vi "Demo.vi"() -> ()   [LabVIEW 2021, in "Ring Buffer Time Series Data.lvlib"]
uses:
  Ring Buffer Time Series Data.lvlib
  SubVIs/Split Values Array.vi
  SubVIs/Replace Values Array Multiple Timestamps.vi
  SubVIs/Rotate Buffer.vi
  SubVIs/Newest Value Index.vi
  SubVIs/empty buffer check.vi
  SubVIs/Replace Values Array One Timestamp.vi
  SubVIs/Enforce array size one timestamp.vi
  SubVIs/Enforce array size multiple timestamps.vi
panel:
  out "empty buffer? (previous)":bool
  out "empty buffer? (latest)":bool
  out "empty buffer?":bool
  out "v-latest 3":u8[](array[numeric])
  out "v-latest 2":u8[](array[numeric])
  out "t-latest 3":u64
  out "t-latest 2":u64
  out "Value changed? 2":bool
  out "Value changed?":bool
  out "v3":u8[](array[numeric])
  out "t3":u64[](array[numeric])
  out "v1":u8[](array[numeric])
  out "t1":u64[](array[numeric])
  out "v-latest":u8[](array[numeric])
  out "t-latest":u64
  out "t2":u64[](array[numeric])
  out "v2":u8[](array[numeric])
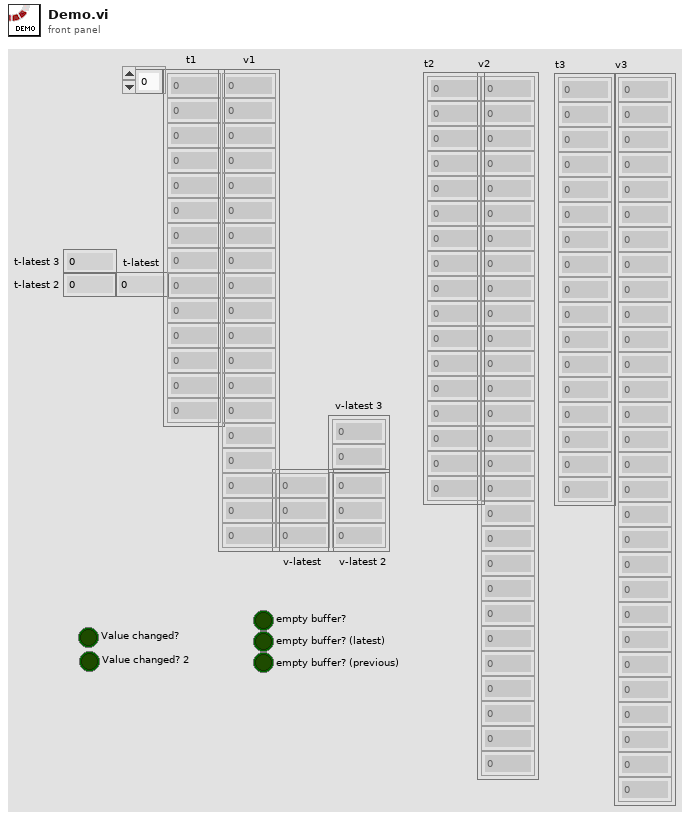
[diagram p1: front panel]
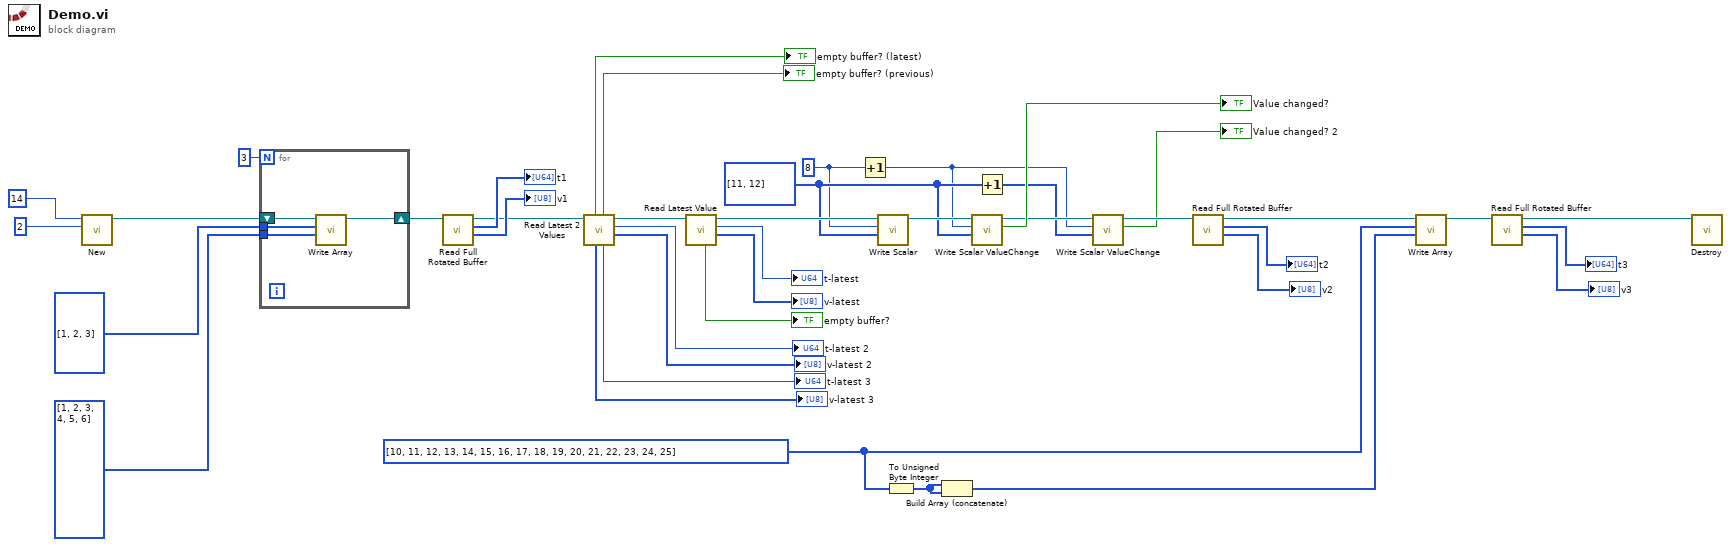
[diagram p0: block diagram]
diagram:
  w26 = u64[] [10, 11, 12, 13, 14, 15, 16, 17, 18, 19, 20, 21, 22, 23, 24, 25] ("Timestamps")
  w14 = u8[] [11, 12] ("Data")
  w12 = u64 8 ("Timestamp")
  n1 = call "New.vi"("#bytes per timestamp"=2 ("#bytes per value"), "Buffer Size (#timestamps)"=14 ("Buffer Size")) -> ("Ring buffer DVR"=w1:refnum<data-value>)  [unwired: 8 in, 1 out]
  n2 = for {
    N: 3 -> [_]
    tunnel: u8[] [1, 2, 3, 4, 5, 6] ("Timestamps") -> [w43]
    tunnel: u64[] [1, 2, 3] ("Timestamps") -> [w41]
    shift-right: [w42] -> w39
    shift-left: w1 -> [w44]
    n3 = call "Write Array.vi"("Data"=w43, "Timestamps"=w41, "Ring buffer DVR in"=w44) -> ("Ring buffer DVR out"=w42:refnum<data-value>)  [unwired: 7 in, 1 out]
  }
  n4 = call "Read Full Rotated Buffer.vi"("Ring buffer DVR in"=w39) -> ("Values"=→"v1":u8[], "Timestamps"=→"t1":u64[], "Ring buffer DVR out"=w10:refnum<data-value>)  [unwired: 5 in, 3 out]
  n5 = call "Read Latest 2 Values.vi"("Ring buffer DVR in"=w10) -> ("Values (latest)"=→"v-latest 2":u8[], "Timestamp (latest)"=→"t-latest 2":u64, "Ring buffer DVR out"=w9:refnum<data-value>, "Timestamp (previous)"=→"t-latest 3":u64, "empty buffer? (previous)"=→"empty buffer? (previous)":bool, "Values (previous)"=→"v-latest 3":u8[], "empty buffer? (latest)"=→"empty buffer? (latest)":bool)  [unwired: 3 in, 1 out]
  n6 = call "Read Latest Value.vi"("Ring buffer DVR in"=w9) -> ("Values"=→"v-latest":u8[], "Timestamp"=→"t-latest":u64, "Ring buffer DVR out"=w34:refnum<data-value>, "empty buffer?"=→"empty buffer?":bool)  [unwired: 6 in, 1 out]
  n7 = Increment(x=w12) -> (x+1=w11:u64)
  n8 = call "Write Scalar.vi"("Data"=w14, "Timestamp"=w12, "Ring buffer DVR in"=w34) -> ("Ring buffer DVR out"=w19:refnum<data-value>)  [unwired: 7 in, 1 out]
  n9 = To Unsigned Byte Integer(number=w26) -> (unsigned 8bit integer=w25:u8[])
  n10 = Build Array (concatenate)(w25, w25) -> (w24:u8[])
  n11 = call "Write Scalar ValueChange.vi"("Data"=w14, "Timestamp"=w11, "Ring buffer DVR in"=w19) -> ("Value changed?"=→"Value changed?":bool, "Ring buffer DVR out"=w17:refnum<data-value>)  [unwired: 6 in, 1 out]
  n12 = Increment(x=w14) -> (x+1=w13:u8[])
  n13 = call "Write Scalar ValueChange.vi"("Data"=w13, "Timestamp"=w11, "Ring buffer DVR in"=w17) -> ("Value changed?"=→"Value changed? 2":bool, "Ring buffer DVR out"=w16:refnum<data-value>)  [unwired: 6 in, 1 out]
  n14 = call "Read Full Rotated Buffer.vi"("Ring buffer DVR in"=w16) -> ("Values"=→"v2":u8[], "Timestamps"=→"t2":u64[], "Ring buffer DVR out"=w29:refnum<data-value>)  [unwired: 5 in, 3 out]
  n15 = call "Write Array.vi"("Data"=w24, "Timestamps"=w26, "Ring buffer DVR in"=w29) -> ("Ring buffer DVR out"=w21:refnum<data-value>)  [unwired: 7 in, 1 out]
  n16 = call "Read Full Rotated Buffer.vi"("Ring buffer DVR in"=w21) -> ("Values"=→"v3":u8[], "Timestamps"=→"t3":u64[], "Ring buffer DVR out"=w20:refnum<data-value>)  [unwired: 5 in, 3 out]
  n17 = call "Destroy.vi"("Ring buffer DVR"=w20) -> ()  [unwired: 10 in, 1 out]
